vi "Configure Output.vi"(0 "VISA resource name":refnum<visa-resource-name>, 1 "Output Real Impedance (0)":dbl format="%#.6g", 2 "Output Reactive Impedance (0.00005)":dbl=5e-05 format="%#.6g", 5 "Output Coupling (0: AC)":i32(ring) items=["AC", "DC"], 7 "Enable Output Impedance Compensation (F: Disable)":bool, 9 "Remote Inhibit (0: Off)":i32(ring) items=["Off", "Latching", "Live"], 11 "error in (no error)":errorcluster, 12 "Enable Discrete Fault Indicator (F: Disable)":bool, 13 "Discrete Fault Indicator Source (0: Off)":i32(ring) items=["Off", "Questionable Summary Bit", "Operation Summary Bit", "Standard Event Summary Bit", "Request Service Summary Bit"], 14 "Trigger Output Source (0: Beginning of Transient Output)":i32(ring) items=["Beginning of Transient Output", "End of Transient Output", "List"]) -> (4 "VISA resource name out":refnum<visa-resource-name>, 15 "error out":errorcluster)   [LabVIEW 2019, in "Agilent 681x Series.lvlib"]
doc: "Configures the output settings of the instrument."
uses:
  <instrlib>/Agilent 681x Series/Agilent 681x Series.lvlib
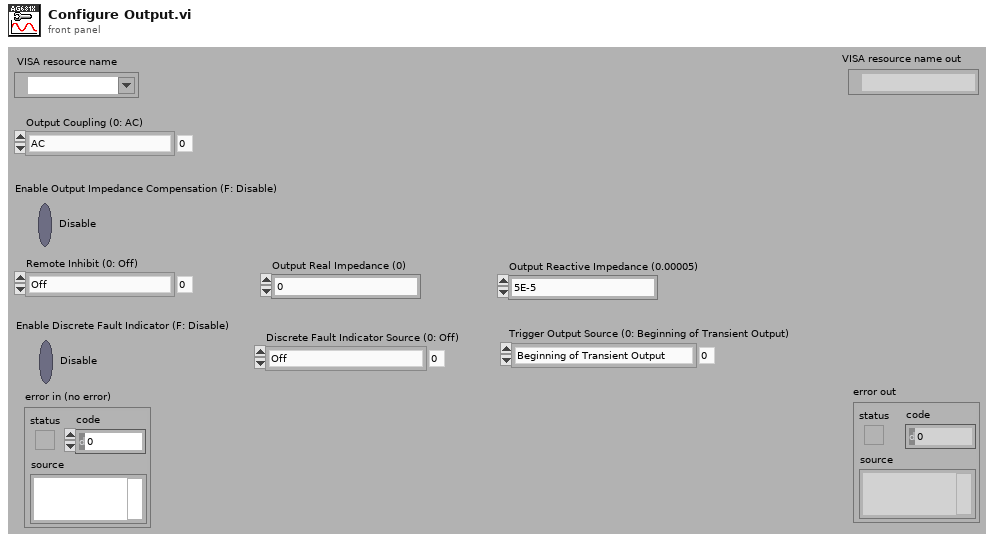
[diagram p1: front panel]
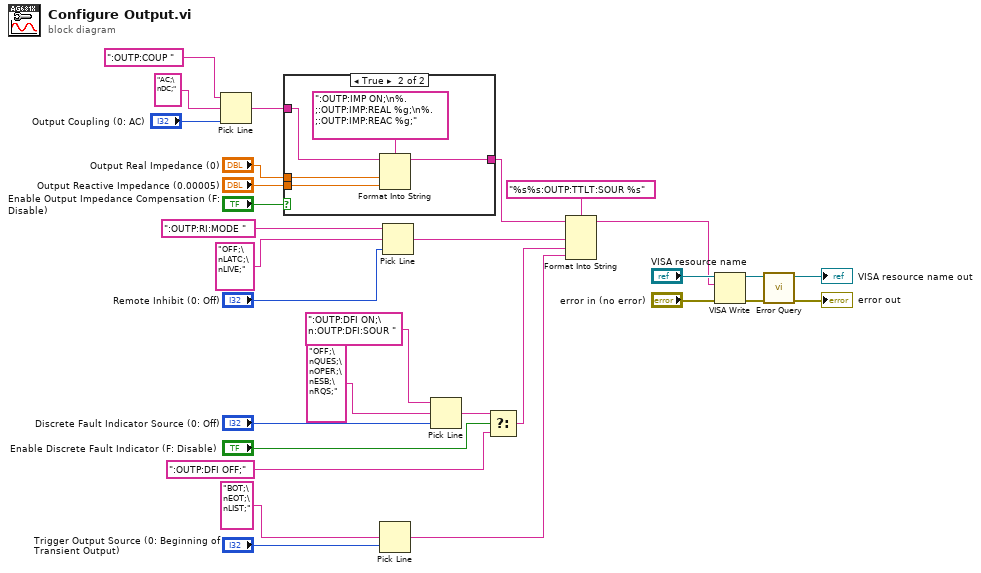
[diagram p0: block diagram]
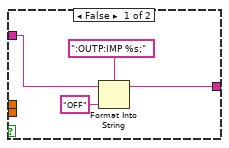
[diagram p2: hidden frame]
diagram:
  n1 = Pick Line(string ("")=":OUTP:COUP ", multi-line string="AC;\nDC;", line index="Output Coupling (0: AC)") -> (output string=w20:string)
  n2 = case shown="True" "Enable Output Impedance Compensation (F: Disable)" {
    tunnel: w20 -> [w34 w37]
    tunnel: "Output Real Impedance (0)" -> [_ w39]
    tunnel: "Output Reactive Impedance (0.00005)" -> [_ w38]
    tunnel: [w31 w35] -> w14
    frame False {
      n3 = Format Into String(format string=":OUTP:IMP %s;", initial string=w34, "OFF" ("input 1")) -> (resulting string=w31:string)  [unwired: 1 in, 1 out]
    }
    frame True {
      n4 = Format Into String(format string=":OUTP:IMP ON;\n%.;:OUTP:IMP:REAL %g;\n%.;:OUTP:IMP:REAC %g;", initial string=w37, w39, w38) -> (resulting string=w35:string)  [unwired: 1 in, 1 out]
    }
  }
  n5 = Pick Line(multi-line string="BOT;\nEOT;\nLIST;", line index="Trigger Output Source (0: Beginning of Transient Output)") -> (output string=w7:string)  [unwired: 1 in]
  n6 = Pick Line(string ("")=":OUTP:RI:MODE ", multi-line string="OFF;\nLATC;\nLIVE;", line index="Remote Inhibit (0: Off)") -> (output string=w13:string)
  n7 = Pick Line(string ("")=":OUTP:DFI ON;\n:OUTP:DFI:SOUR ", multi-line string="OFF;\nQUES;\nOPER;\nESB;\nRQS;", line index="Discrete Fault Indicator Source (0: Off)") -> (output string=w3:string)
  n8 = Select(t=w3, s="Enable Discrete Fault Indicator (F: Disable)", f=":OUTP:DFI OFF;") -> (s? t:f=w1:string)
  n9 = Format Into String(format string="%s%s:OUTP:TTLT:SOUR %s", initial string=w14, w13, w1, w7) -> (resulting string=w10:string)  [unwired: 1 in, 1 out]
  n10 = VISA Write(VISA resource name="VISA resource name", write buffer=w10, error in (no error)="error in (no error)") -> (VISA resource name out=w28:refnum<visa-resource-name>, error out=w27:errorcluster)  [unwired: 1 out]
  n11 = call <instrlib>:"Error Query.vi"("error in (no error)"=w27, "VISA resource name"=w28) -> ("error out"=→"error out":errorcluster, "VISA resource name out"=→"VISA resource name out":refnum<visa-resource-name>)  [unwired: 6 in, 2 out]
